vi "Find Subcrystal.vi"(10 "Base Atom":i32, 11 "Atomic Structure":T1={"Structure Name"="Gamm8", "Lattice vector a"=[4.675927601962877, 0.0, 0.0], "Lattice vector b"=[0.0, 8.100295396595834, -6.14689389815e-05], "Lattice vector c"=[0.0, -8.67870405793e-05, 11.452598090719311], "Atoms Array"=[{"Atom Name"="Cd", "Positions (Direct)"=[[0.0, 2.2797955771e-06, 0.2499966378910753], [0.5000009999999975, 0.5000032797955746, 0.2499966378910753], [0.0, 0.3333362797955778, 0.583330637891076], [0.5000009999999975, 0.8333372797955753, 0.583330637891076], [0.5000009999999975, 0.1666692797955739, 0.9166636378910721], [0.0, 0.6666702797955785, 0.9166636378910721]], "Positions (Cartesian)"=[[0.0, -3.2294507389786483e-06, 2.863111017657439], [2.3379684769090283, 4.050152569142555, 2.8630802831264797], [0.0, 2.700071707206758, 6.680630859941972], [2.3379684769090283, 6.750227505800051, 6.6806001254110114], [2.3379684769090283, 1.349990845357691, 10.49816998415932], [0.0, 5.400146643951042, 10.49813924962836]]}, {"Atom Name"="Te", "Positions (Direct)"=[[0.0, 0.3333317202044236, 0.3333363621089279], [0.5000009999999975, 0.8333327202044211, 0.3333363621089279], [0.5000009999999975, 0.1666647202044197, 0.6666703621089215], [0.0, 0.6666657202044243, 0.6666703621089215], [0.0, -2.2797955771e-06, 3.3621089247e-06], [0.5000009999999975, 0.4999987202044204, 3.3621089247e-06]], "Positions (Cartesian)"=[[0.0, 2.700056469434878, 3.8175468947088587], [2.3379684769090283, 6.7502122680281715, 3.8175161601778993], [2.3379684769090283, 1.3499756074990243, 7.635097471524269], [0.0, 5.400131406092375, 7.63506673699331], [0.0, -1.8467309405846353e-05, 3.850502238842479e-05], [2.3379684769090283, 4.050137331283887, 7.770491428735963e-06]]}], "# of atoms"=12} {"Atoms Array"."Positions (Cartesian)" format="%#_4f"; "Atoms Array"."Positions (Direct)" format="%#_3f"}) -> (0 "Base Atom Position (Cartesian)":dbl[](array[numeric]), 2 "Supercell Positions":dbl[][](array[numeric])=[[1.0, 0.0, 0.0], [0.0, 1.0, 0.0], [1.0, 1.0, 0.0], [-1.0, 2.0, 1.0], [0.0, 2.0, -0.0]], 3 "Subcrystal":T1={"Structure Name"="Gamm8 Subcrystal", "Lattice vector a"=[2.3379684769090283, 4.050155798593294, -3.073453095936429e-05], "Lattice vector b"=[0.0, 2.7000749366574968, 3.8175198422845327], "Lattice vector c"=[4.675927601962877, 0.0, 0.0], "Atoms Array"=[{"Atom Name"="Cd", "Positions (Direct)"=[[0.0, 2.2797955771e-06, 0.2499966378910753]], "Positions (Cartesian)"=[[0.0, -3.2294507389786483e-06, 2.863111017657439]]}, {"Atom Name"="Te", "Positions (Direct)"=[[0.0, -2.2797955771e-06, 3.3621089247e-06]], "Positions (Cartesian)"=[[0.0, -1.5237858666867705e-05, -2.8630725126350507]]}], "# of atoms"=2} {"Atoms Array"."Positions (Cartesian)" format="%#_4f"; "Atoms Array"."Positions (Direct)" format="%#_4f"})   [LabVIEW 2010]
uses:
  <vilib>/Analysis/baseanly.llb/Real Inverse Matrix.vi
  <vilib>/Analysis/baseanly.llb/A x Vector.vi
  <vilib>/Analysis/_algsub.llb/Real Vector Norm.vi
  <vilib>/Analysis/NI_AALPro.lvlib
  <vilib>/Analysis/NI_AALBase.lvlib
panel:
  out "norm":dbl
  out "A x Vector 2":dbl[][](array[numeric])
  out "Remaining Indicies":i32[](array[numeric])
  out "A x Vector":dbl[][](array[numeric])
  out "Recovered Positions":dbl[][](array[numeric])=[[0.33811863359999994, 1.0281858879, 1.8934606114], [4.9201686336, 1.0281858879, 1.8934606114], [2.629143633599999, 4.9963608879, 1.8934606114], [7.2111936336, 4.9963608879, 1.8934606114], [2.6155716014999992, 2.34227878455, 5.7830199243000004], [7.1976216015, 2.34227878455, 5.7830199243000004], [0.32454660149999826, 6.310453784549999, 5.7830199243000004], [4.906596601499999, 6.310453784549999, 5.7830199243000004]]
  in  "Integer Threshold":dbl=0.001
  out "Atoms Array":T2(array[cluster])=[{"Atom Name"="", "Positions (Direct)"=[[0.036896, 0.129554, 0.035254], [0.536896, 0.129554, 0.035254], [0.286896, 0.629554, 0.035254], [0.786896, 0.629554, 0.035254], [0.285415, 0.295133, 0.107673], [0.785415, 0.295133, 0.107673], [0.035415, 0.795133, 0.107673], [0.535415, 0.795133, 0.107673], [0.033615, 0.463308, 0.180101], [0.533615, 0.463308, 0.180101], [0.283615, 0.963308, 0.180101], [0.783615, 0.963308, 0.180101], [0.030844, 0.131453, 0.252535], [0.530844, 0.131453, 0.252535], [0.280844, 0.631453, 0.252535], [0.780844, 0.631453, 0.252535], [0.278379, 0.302058, 0.324923], [0.778379, 0.302058, 0.324923], [0.028379, 0.802058, 0.324923], [0.528379, 0.802058, 0.324923], [0.031198, 0.471844, 0.397363], [0.531198, 0.471844, 0.397363], [0.281198, 0.971844, 0.397363], [0.781198, 0.971844, 0.397363], [0.03247, 0.140643, 0.469814], [0.53247, 0.140643, 0.469814], [0.28247, 0.640643, 0.469814], [0.78247, 0.640643, 0.469814], [0.284308, 0.303948, 0.542263], [0.784308, 0.303948, 0.542263], [0.034308, 0.803948, 0.542263], [0.534308, 0.803948, 0.542263], [0.035944, 0.468219, 0.614701], [0.535944, 0.468219, 0.614701], [0.285944, 0.968219, 0.614701], [0.785944, 0.968219, 0.614701], [0.037813, 0.131858, 0.687216], [0.537813, 0.131858, 0.687216], [0.787813, 0.631858, 0.687216], [0.287813, 0.631858, 0.687216], [0.038238, 0.463759, 0.759817], [0.538238, 0.463759, 0.759817], [0.288238, 0.963758, 0.759817], [0.788238, 0.963758, 0.759817], [0.038639, 0.130134, 0.831025], [0.538639, 0.130134, 0.831025], [0.288639, 0.630134, 0.831025], [0.788639, 0.630134, 0.831025], [0.285712, 0.295024, 0.89873], [0.785712, 0.295024, 0.89873], [0.035712, 0.795024, 0.89873], [0.535712, 0.795024, 0.89873], [0.032596, 0.464879, 0.966384], [0.532596, 0.464879, 0.966384], [0.282596, 0.964879, 0.966384], [0.782596, 0.964879, 0.966384]], "Positions (Cartesian)"=[[0.33811863359999994, 1.0281858879, 1.8934606114], [4.9201686336, 1.0281858879, 1.8934606114], [2.6291436335999996, 4.9963608879, 1.8934606114], [7.2111936336, 4.9963608879, 1.8934606114], [2.6155716014999997, 2.34227878455, 5.7830199243000004], [7.197621601499999, 2.34227878455, 5.7830199243000004], [0.3245466015, 6.31045378455, 5.7830199243000004], [4.9065966014999995, 6.31045378455, 5.7830199243000004], [0.30805122149999997, 3.6769744458, 9.673062619100001], [4.890101221499999, 3.6769744458, 9.673062619100001], [2.5990762215, 7.6451494458, 9.673062619100001], [7.1811262215, 7.6451494458, 9.673062619100001], [0.2826575004, 1.04325701655, 13.5634275685], [4.8647075004, 1.04325701655, 13.5634275685], [2.5736825004, 5.011432016550001, 13.5634275685], [7.155732500399999, 5.011432016550001, 13.5634275685], [2.5510929938999998, 2.3972380083, 17.4513218993], [7.1331429939, 2.3972380083, 17.4513218993], [0.2600679939, 6.3654130083, 17.4513218993], [4.8421179939000005, 6.3654130083, 17.4513218993], [0.28590159179999997, 3.7447191294, 21.3420091033], [4.867951591799999, 3.7447191294, 21.3420091033], [2.5769265918, 7.7128941294, 21.3420091033], [7.158976591799999, 7.7128941294, 21.3420091033], [0.29755832699999996, 1.11619207305, 25.2332871074], [4.879608327, 1.11619207305, 25.2332871074], [2.588583327, 5.08436707305, 25.2332871074], [7.170633327, 5.08436707305, 25.2332871074], [2.6054269428, 2.4122377098, 29.124457693300002], [7.1874769428, 2.4122377098, 29.124457693300002], [0.31440194279999994, 6.3804127098, 29.124457693300002], [4.8964519428, 6.3804127098, 29.124457693300002], [0.32939441039999995, 3.71594986065, 33.0150374791], [4.9114444104, 3.71594986065, 33.0150374791], [2.6204194104, 7.684124860650001, 33.0150374791], [7.202469410399999, 7.684124860650001, 33.0150374791], [0.3465221133, 1.0464712383, 36.909752865600005], [4.9285721133, 1.0464712383, 36.909752865600005], [7.2195971133, 5.0146462383, 36.909752865600005], [2.6375471132999997, 5.0146462383, 36.909752865600005], [0.3504168558, 3.6805537396499997, 40.809087234699994], [4.9324668557999995, 3.6805537396499997, 40.809087234699994], [2.6414418557999997, 7.6487208033, 40.809087234699994], [7.2234918558, 7.6487208033, 40.809087234699994], [0.35409165989999997, 1.0327889709, 44.6336048275], [4.9361416599, 1.0327889709, 44.6336048275], [2.6451166599, 5.0009639709, 44.6336048275], [7.227166659899999, 5.0009639709, 44.6336048275], [2.6182933392, 2.3414137224, 48.269979443000004], [7.200343339199999, 2.3414137224, 48.269979443000004], [0.3272683392, 6.3095887224, 48.269979443000004], [4.9093183391999995, 6.3095887224, 48.269979443000004], [0.29871300359999997, 3.6894424516499997, 51.9036148944], [4.880763003599999, 3.6894424516499997, 51.9036148944], [2.5897380036, 7.65761745165, 51.9036148944], [7.171788003599999, 7.65761745165, 51.9036148944]]}, {"Atom Name"="", "Positions (Direct)"=[[0.286795, 0.296109, 0.054458], [0.786795, 0.296109, 0.054458], [0.036795, 0.796109, 0.054458], [0.536795, 0.796109, 0.054458], [0.035258, 0.462031, 0.126878], [0.535258, 0.462031, 0.126878], [0.285258, 0.962031, 0.126878], [0.785258, 0.962031, 0.126878], [0.033445, 0.130094, 0.199309], [0.533445, 0.130094, 0.199309], [0.283445, 0.630094, 0.199309], [0.783445, 0.630094, 0.199309], [0.280766, 0.298203, 0.27171], [0.780766, 0.298203, 0.27171], [0.030766, 0.798203, 0.27171], [0.530766, 0.798203, 0.27171], [0.028505, 0.468822, 0.344121], [0.528505, 0.468822, 0.344121], [0.278505, 0.968822, 0.344121], [0.778505, 0.968822, 0.344121], [0.03126, 0.138635, 0.416572], [0.53126, 0.138635, 0.416572], [0.28126, 0.638635, 0.416572], [0.78126, 0.638635, 0.416572], [0.282556, 0.307128, 0.489026], [0.782556, 0.307128, 0.489026], [0.032556, 0.807128, 0.489026], [0.532556, 0.807128, 0.489026], [0.034374, 0.470438, 0.56147], [0.534374, 0.470438, 0.56147], [0.284374, 0.970438, 0.56147], [0.784374, 0.970438, 0.56147], [0.035964, 0.134698, 0.633895], [0.535964, 0.134698, 0.633895], [0.285964, 0.634698, 0.633895], [0.785964, 0.634698, 0.633895], [0.037794, 0.465111, 0.706493], [0.537794, 0.465111, 0.706493], [0.787794, 0.965111, 0.706493], [0.287794, 0.965111, 0.706493], [0.038181, 0.130274, 0.779081], [0.538181, 0.130274, 0.779081], [0.288181, 0.630273, 0.779081], [0.788181, 0.630273, 0.779081], [0.288548, 0.296604, 0.847022], [0.788548, 0.296604, 0.847022], [0.038548, 0.796604, 0.847022], [0.538548, 0.796604, 0.847022], [0.035661, 0.461866, 0.914714], [0.535661, 0.461866, 0.914714], [0.285661, 0.961866, 0.914714], [0.785661, 0.961866, 0.914714], [0.032517, 0.131341, 0.982331], [0.532517, 0.131341, 0.982331], [0.282517, 0.631341, 0.982331], [0.782517, 0.631341, 0.982331]], "Positions (Cartesian)"=[[2.6282180595, 2.35002466215, 2.9248901678], [7.2102680595, 2.35002466215, 2.9248901678], [0.3371930595, 6.31819966215, 2.9248901678], [4.9192430595, 6.31819966215, 2.9248901678], [0.32310783779999996, 3.66683972685, 6.814503189799999], [4.9051578378, 3.66683972685, 6.814503189799999], [2.6141328378, 7.63501472685, 6.814503189799999], [7.1961828377999995, 7.63501472685, 6.814503189799999], [0.3064933245, 1.0324715168999998, 10.704707011899998], [4.8885433245, 1.0324715168999998, 10.704707011899998], [2.5975183244999998, 5.000646516900001, 10.704707011899998], [7.179568324499999, 5.000646516900001, 10.704707011899998], [2.5729677006, 2.36664337905, 14.593299561], [7.155017700599999, 2.36664337905, 14.593299561], [0.2819427006, 6.33481837905, 14.593299561], [4.863992700599999, 6.33481837905, 14.593299561], [0.2612226705, 3.7207354797, 18.4824292011], [4.843272670499999, 3.7207354797, 18.4824292011], [2.5522476705, 7.6889104797, 18.4824292011], [7.1342976705, 7.6889104797, 18.4824292011], [0.286469766, 1.1002558822500002, 22.3737072052], [4.8685197659999995, 1.1002558822500002, 22.3737072052], [2.577494766, 5.0684308822499995, 22.3737072052], [7.159544765999999, 5.0684308822499995, 22.3737072052], [2.5893714396, 2.4374753028000002, 26.2651463366], [7.1714214396, 2.4374753028000002, 26.2651463366], [0.2983464396, 6.4056503028, 26.2651463366], [4.8803964396, 6.4056503028, 26.2651463366], [0.3150067734, 3.7335606213, 30.156048377], [4.8970567734, 3.7335606213, 30.156048377], [2.6060317734, 7.7017356213, 30.156048377], [7.1880817733999995, 7.7017356213, 30.156048377], [0.3295776924, 1.0690104723, 34.045929944499996], [4.9116276924, 1.0690104723, 34.045929944499996], [2.6206026924, 5.0371854723, 34.045929944499996], [7.202652692399999, 5.0371854723, 34.045929944499996], [0.3463479954, 3.69128368485, 37.9451031863], [4.928397995399999, 3.69128368485, 37.9451031863], [7.2194229953999995, 7.659458684850001, 37.9451031863], [2.6373729954, 7.659458684850001, 37.9451031863], [0.34989450209999995, 1.0339000599000001, 41.843739337100004], [4.9319445020999995, 1.0339000599000001, 41.843739337100004], [2.6409195021, 5.00206712355, 41.843739337100004], [7.2229695021, 5.00206712355, 41.843739337100004], [2.6442827268, 2.3539531553999997, 45.4927893002], [7.2263327268, 2.3539531553999997, 45.4927893002], [0.35325772679999995, 6.3221281554, 45.4927893002], [4.9353077268, 6.3221281554, 45.4927893002], [0.3268009701, 3.6655302291, 49.1284656974], [4.9088509701000005, 3.6655302291, 49.1284656974], [2.6178259700999997, 7.6337052291, 49.1284656974], [7.1998759701, 7.6337052291, 49.1284656974], [0.29798903969999996, 1.04236814535, 52.760113912099996], [4.8800390397, 1.04236814535, 52.760113912099996], [2.5890140397, 5.010543145350001, 52.760113912099996], [7.1710640397, 5.010543145350001, 52.760113912099996]]}]
  # "Need not be equal since the Cd and Te aren't paired"
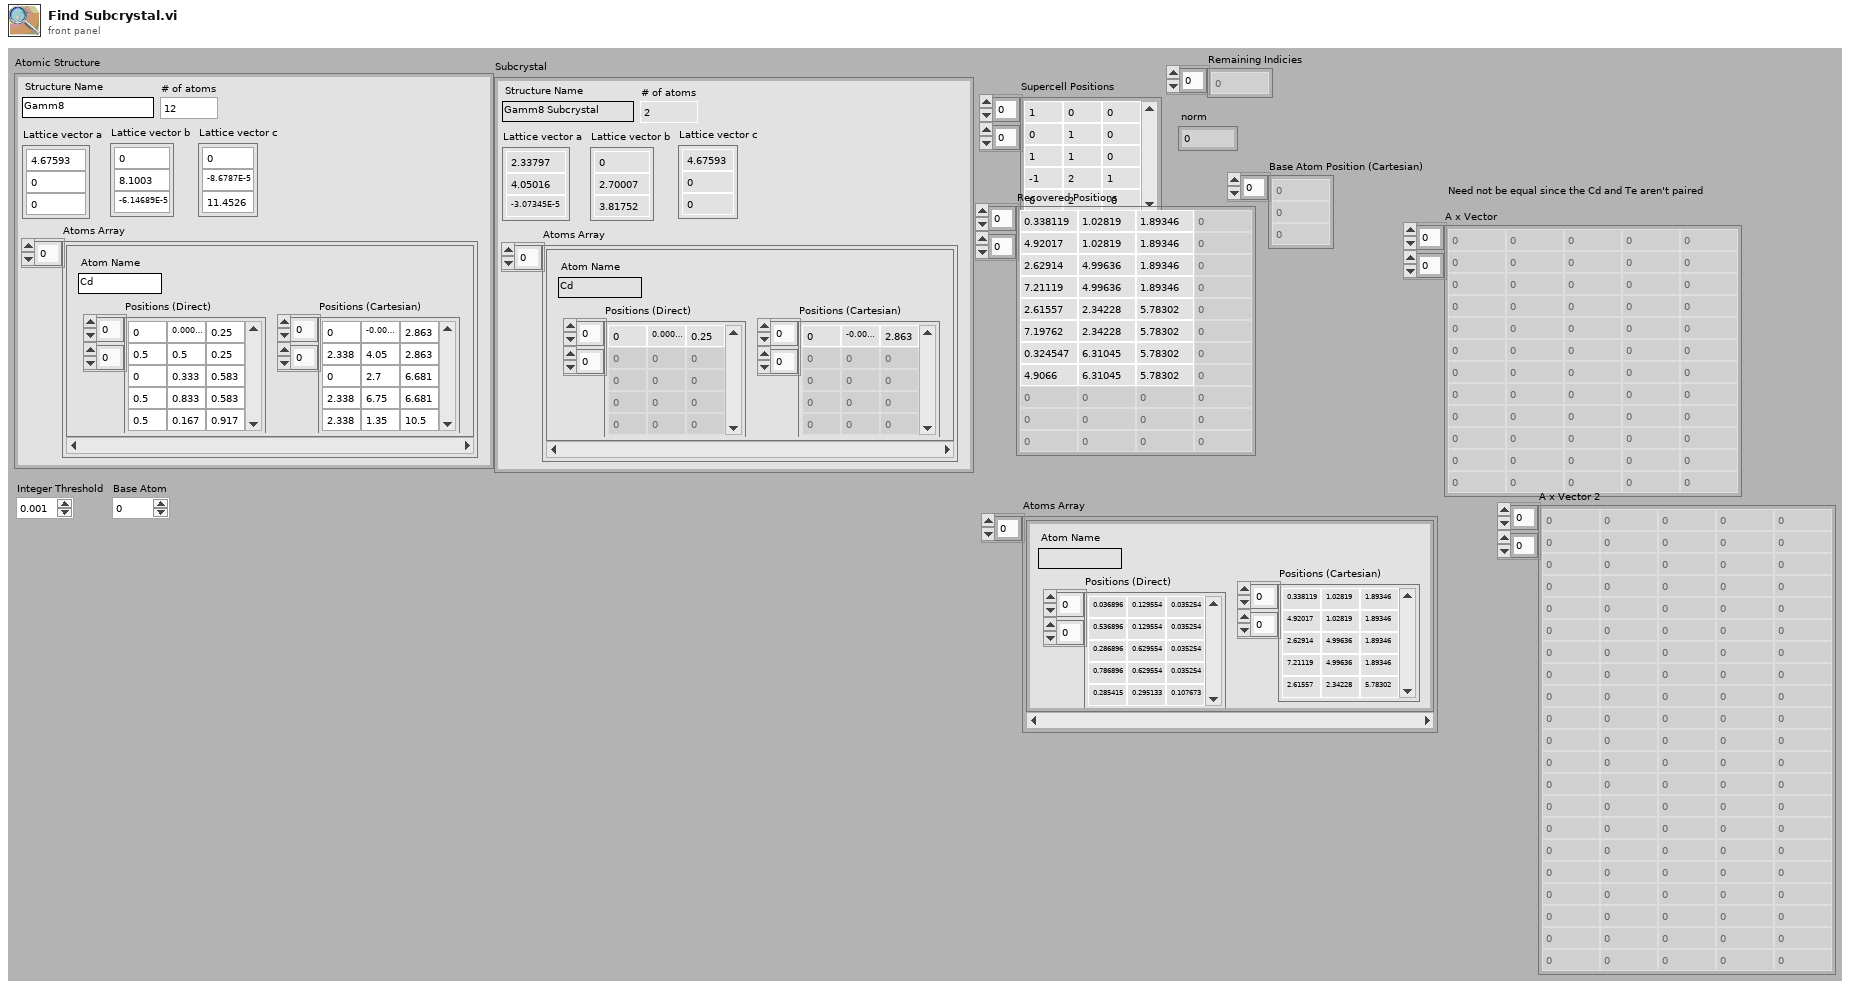
[diagram p1: front panel]
types:
  T1 = cluster{"Structure Name":string, "Lattice vector a":dbl[], "Lattice vector b":dbl[], "Lattice vector c":dbl[], "Atoms Array":cluster{"Atom Name":string, "Positions (Direct)":dbl[][], "Positions (Cartesian)":dbl[][]}[], "# of atoms":i32}
  T2 = cluster{"Atom Name":string, "Positions (Direct)":dbl[][], "Positions (Cartesian)":dbl[][]}[]
  T3 = cluster{"Atom Name":string, "Positions (Direct)":dbl[][], "Positions (Cartesian)":dbl[][]}
  T4 = typedef "NI_Matrix.lvlib/RealMatrix.ctl" = dbl[][]
  T5 = cluster{string, dbl[], dbl[], dbl[], cluster{"Atom Name":string, dbl[][], dbl[][]}[], "index (row)":i32}
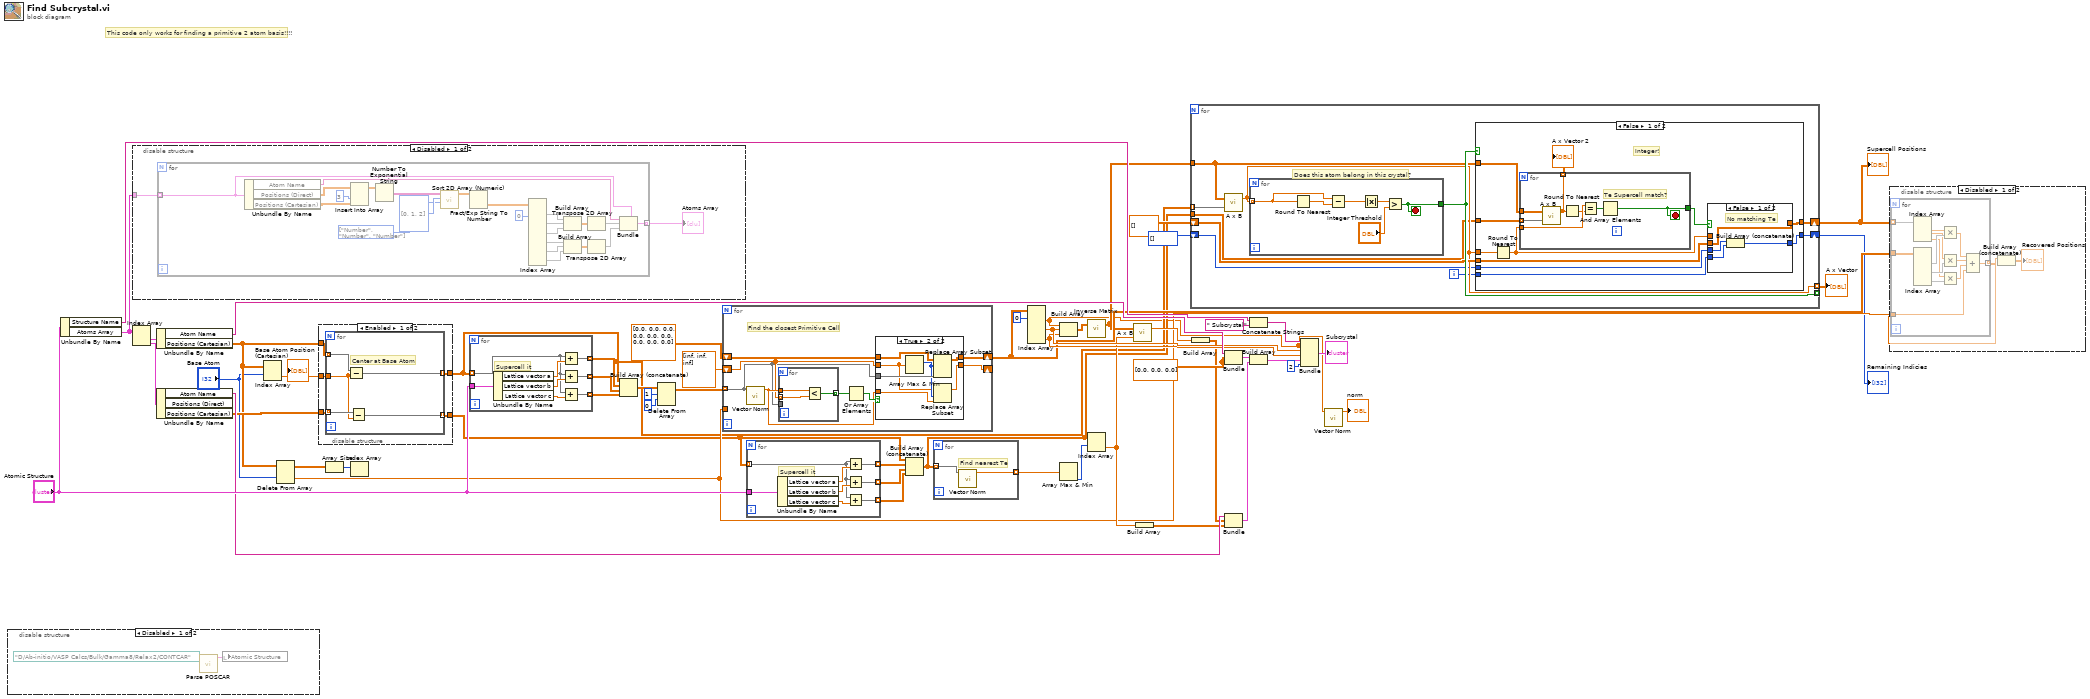
[diagram p0: block diagram]
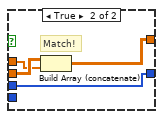
[diagram p5: hidden frame]
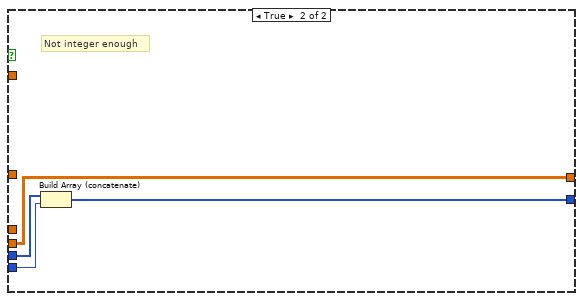
[diagram p6: hidden frame]
diagram:
  w22 = dbl[][] [[0.0, 0.0, 0.0]]
  # "This code only works for finding a primitive 2 atom basis!!!!"
  n1 = disable-structure shown="Disabled" {
    frame Disabled {
      n2 = call "Parse POSCAR.vi"("POSCAR File"=path "D:/Ab-initio/VASP Calcs/Bulk/Gamma8/Relax2/CONTCAR") -> ("Structure"=w58:T1)  [unwired: 7 in, 3 out]
      n3 = local write "Atomic Structure"(w58) -> ()
    }
    frame Enabled {
    }
  }
  n4 = Unbundle By Name("Atomic Structure") -> ("Structure Name"=w53:string, "Atoms Array"=w56:T2)
  n5 = disable-structure shown="Disabled" {
    disable-tunnel: w56 -> [w59 _]
    frame Disabled {
      n6 = for {
        tunnel: w59 -> [w61] mode=indexing
        tunnel: [w71] -> w60 mode=indexing
        w82 = enum16{"String", "Number", "Date-Time"}[] [enum."Number", enum."Number", enum."Number"] items=["String", "Number", "Date-Time"] ("Sort by Datatype Array")
        n7 = Unbundle By Name(w61) -> ("Atom Name"=w72:string, "Positions (Direct)"=w70:dbl[][], "Positions (Cartesian)"=w69:dbl[][])
        n8 = Insert Into Array(array=w70, index (col)=3 ("disabled index (col)"), new element=w69) -> (w67:dbl[][])  [unwired: 1 in]
        n9 = Number To Exponential String(number=w67) -> (E-format string=w81:string[][])  [unwired: 3 in]
        n10 = call "Sort 2D Array (Numeric).vi"(9:w82, "Sort by Cols"=i32[] [0, 1, 2], "Input Array"=w81) -> ("Output Array"=w80:dbl[][])  [unwired: 8 in]
        n11 = Fract/Exp String To Number(string=w80) -> (number=w66:dbl[][])  [unwired: 3 in, 1 out]
        n12 = Index Array(array=w66, index (col) #1=0 ("disabled index (col)")) -> (element #1=w78:dbl[], element #2=w77:dbl[], element #3=w76:dbl[], element #4=w75:dbl[], element #5=w74:dbl[], element #6=w73:dbl[])  [unwired: 11 in]
        n13 = Build Array(w78, w77, w76) -> (w65:dbl[][])
        n14 = Build Array(w75, w74, w73) -> (w63:dbl[][])
        n15 = Transpose 2D Array(2D array=w65) -> (transposed array=w64:dbl[][])
        n16 = Transpose 2D Array(2D array=w63) -> (transposed array=w62:dbl[][])
        n17 = Bundle(cluster=w61, "Atom Name"=w72, "Positions (Direct)"=w64, "Positions (Cartesian)"=w62) -> (w71:T3)
      }
      "Atoms Array" <- w60
    }
    frame Enabled {
    }
  }
  n18 = Index Array(array=w56) -> (element #1=w55:T3, element #2=w51:T3)  [unwired: 2 in]
  n19 = Unbundle By Name(w55) -> ("Atom Name"=w52:string, "Positions (Cartesian)"=w14:dbl[][])
  n20 = Unbundle By Name(w51) -> ("Atom Name"=w50:string, "Positions (Cartesian)"=w15:dbl[][])  [unwired: 1 out]
  n21 = Index Array(array=w14, index (row)="Base Atom") -> (element=w12:dbl[])  [unwired: 1 in]
  "Base Atom Position (Cartesian)" <- w12
  n22 = Delete From Array(array=w14, index (row)="Base Atom") -> (deleted portion=w16:dbl[], array with subset deleted=w31:dbl[][])  [unwired: 2 in]
  n23 = disable-structure shown="Enabled" {
    disable-tunnel: w15 -> [w88 w94]
    disable-tunnel: w14 -> [w87 w95]
    disable-tunnel: w12 -> [w86 _]
    disable-tunnel: [w85 w95] -> w7
    disable-tunnel: [w84 w94] -> w6
    frame Enabled {
      n24 = for {
        tunnel: w87 -> [w93] mode=indexing
        tunnel: w86 -> [w91]
        tunnel: w88 -> [w92] mode=indexing
        tunnel: [w90] -> w84 mode=indexing
        tunnel: [w89] -> w85 mode=indexing
        # "Center at Base Atom"
        n25 = Subtract(x=w93, y=w91) -> (x-y=w89:dbl[])
        n26 = Subtract(x=w92, y=w91) -> (x-y=w90:dbl[])
      }
    }
    frame Disabled {
    }
  }
  n27 = Array Size(array=w31) -> (size(s)=w43:i32[])
  n28 = Index Array(array=w43) -> ()  [unwired: 1 in, 1 out]
  n29 = for {
    tunnel: w7 -> [w100] mode=indexing
    tunnel: "Atomic Structure" -> [w103]
    tunnel: [w98] -> w47 mode=indexing
    tunnel: [w97] -> w46 mode=indexing
    tunnel: [w96] -> w45 mode=indexing
    # "Supercell it"
    n30 = Unbundle By Name(w103) -> ("Lattice vector a"=w102:dbl[], "Lattice vector b"=w101:dbl[], "Lattice vector c"=w99:dbl[])
    n31 = Add(x=w100, y=w102) -> (x+y=w98:dbl[])
    n32 = Add(x=w100, y=w101) -> (x+y=w97:dbl[])
    n33 = Add(x=w100, y=w99) -> (x+y=w96:dbl[])
  }
  n34 = Build Array (concatenate)(w7, w47, w46, w45) -> (w11:dbl[][])
  n35 = Delete From Array(array=w11, length=1, index (row)=0) -> (array with subset deleted=w8:dbl[][])  [unwired: 1 in, 1 out]
  n36 = for {
    tunnel: w16 -> [_]
    tunnel: w8 -> [w104] mode=indexing
    shift-right: [w105] -> _
    shift-left: dbl[] [inf, inf, inf] -> [w106]
    shift-right: [w108] -> w32
    shift-left: dbl[][] [[0.0, 0.0, 0.0], [0.0, 0.0, 0.0], [0.0, 0.0, 0.0]] -> [w109]
    # "Find the closest Primitive Cell"
    n37 = call-poly <vilib>:"Vector Norm.vi"("Input Vector"=w104) -> ("norm"=w107:dbl)  [unwired: 9 in, 1 out]
    n38 = for {
      tunnel: w107 -> [w123]
      tunnel: w106 -> [w122] mode=indexing
      tunnel: w104 -> [_]
      tunnel: [w121] -> w111 mode=indexing
      n39 = Less?(x=w123, y=w122) -> (x < y?=w121:bool)
    }
    n40 = Or Array Elements(Boolean array=w111) -> (logical OR=w110:bool)
    n41 = case shown="True" w110 {
      tunnel: [w113 w120] -> w108
      tunnel: w109 -> [w113 w119]
      tunnel: w104 -> [_ w118]
      tunnel: w106 -> [w112 w114]
      tunnel: w107 -> [_ w117]
      tunnel: [w112 w116] -> w105
      frame False {
      }
      frame True {
        n42 = Array Max & Min(array=w114) -> (max index (indices)=w115:i32)  [unwired: 3 out]
        n43 = Replace Array Subset(array=w119, new element=w118, index (row)=w115) -> (w120:dbl[][])  [unwired: 1 in]
        n44 = Replace Array Subset(array=w114, new element=w117, index=w115) -> (w116:dbl[])
      }
    }
  }
  n45 = for {
    tunnel: w6 -> [w128] mode=indexing
    tunnel: "Atomic Structure" -> [w131]
    tunnel: [w126] -> w30 mode=indexing
    tunnel: [w125] -> w29 mode=indexing
    tunnel: [w124] -> w28 mode=indexing
    # "Supercell it"
    n46 = Unbundle By Name(w131) -> ("Lattice vector a"=w130:dbl[], "Lattice vector b"=w129:dbl[], "Lattice vector c"=w127:dbl[])
    n47 = Add(x=w128, y=w130) -> (x+y=w126:dbl[])
    n48 = Add(x=w128, y=w129) -> (x+y=w125:dbl[])
    n49 = Add(x=w128, y=w127) -> (x+y=w124:dbl[])
  }
  n50 = Build Array (concatenate)(w6, w30, w29, w28) -> (w5:dbl[][])
  n51 = for {
    tunnel: w5 -> [w132] mode=indexing
    tunnel: [w133] -> w27 mode=indexing
    # "Find nearest Te"
    n52 = call-poly <vilib>:"Vector Norm.vi"("Input Vector"=w132) -> ("norm"=w133:dbl)  [unwired: 9 in, 1 out]
  }
  n53 = Index Array(array=w32, index (row) #1=0 ("index (row)")) -> (element #1=w2:dbl[], element #2=w34:dbl[], element #3=w33:dbl[])  [unwired: 5 in]
  n54 = Build Array(w2, w34, w33) -> (w21:T4)
  n55 = Array Max & Min(array=w27) -> (min index (indices)=w25:i32)  [unwired: 3 out]
  n56 = call-poly <vilib>:"Inverse Matrix.vi"("Input Matrix"=w21) -> ("Inverse Matrix"=w17:T4)  [unwired: 1 in, 1 out]
  n57 = Index Array(array=w5, index (row)=w25) -> (element=w20:dbl[])  [unwired: 1 in]
  n58 = call-poly <vilib>:"A x B.vi"("Vector"=w20, "A"=w17) -> ("A x Vector"=w19:dbl[])  [unwired: 1 out]
  n59 = Build Array(w20) -> (w26:dbl[][])
  n60 = for {
    tunnel: w17 -> [w137]
    shift-right: [w143] -> w35
    shift-left: dbl[][] [] -> [w141]
    tunnel: [w142] -> _ mode=indexing
    tunnel: w7 -> [w140] mode=indexing
    tunnel: [w139] -> w23 mode=indexing
    tunnel: w5 -> [w138]
    shift-right: [w135] -> w3
    shift-left: i32[] [] -> [w134]
    i -> [w136]
    # "Does this atom belong in this crystal?"
    n61 = call-poly <vilib>:"A x B.vi"("Vector"=w140, "A"=w137) -> ("A x Vector"=w139:dbl[])  [unwired: 1 out]
    n62 = for {
      tunnel: [w174] -> w142
      tunnel: w139 -> [w176] mode=indexing
      stop <- w174 stop-if-true
      n63 = Round To Nearest(number=w176) -> (nearest integer value=w175:dbl)
      n64 = Subtract(x=w176, y=w175) -> (x-y=w178:dbl)
      n65 = Absolute Value(x=w178) -> (abs(x)=w179:dbl)
      n66 = Greater?(x=w179, y="Integer Threshold") -> (0:w174:bool)
    }
    n67 = case shown="False" w142 {
      tunnel: [w150 w173] -> w143
      tunnel: w141 -> [w151 w173]
      tunnel: w139 -> [w154 _]
      tunnel: w138 -> [w153 _]
      tunnel: w137 -> [w152 _]
      tunnel: w136 -> [w148 w171]
      tunnel: [w147 w170] -> w135
      tunnel: w134 -> [w146 w172]
      frame False {
        # "Integer!"
        n68 = Round To Nearest(number=w154) -> (nearest integer value=w149:dbl[])
        n69 = for {
          tunnel: w149 -> [w169]
          tunnel: w153 -> [w168] mode=indexing
          tunnel: w152 -> [w167]
          tunnel: [w164] -> w145
          tunnel: [w163] -> w144 mode=indexing
          stop <- w164 stop-if-true
          # "Te Supercell match?"
          n70 = call-poly <vilib>:"A x B.vi"("Vector"=w168, "A"=w167) -> ("A x Vector"=w163:dbl[])  [unwired: 1 out]
          n71 = Round To Nearest(number=w163) -> (nearest integer value=w166:dbl[])
          n72 = Equal?(x=w169, y=w166) -> (x = y?=w165:bool[])
          n73 = And Array Elements(Boolean array=w165) -> (logical AND=w164:bool)
        }
        "A x Vector 2" <- w144
        n74 = case shown="False" w145 {
          tunnel: w151 -> [w158 w162]
          tunnel: [w158 w161] -> w150
          tunnel: w149 -> [_ w160]
          tunnel: w148 -> [w157 _]
          tunnel: [w156 w159] -> w147
          tunnel: w146 -> [w155 w159]
          frame False {
            # "No matching Te"
            n75 = Build Array (concatenate)(w155, w157) -> (w156:i32[])
          }
          frame True {
            # "Match!"
            n76 = Build Array (concatenate)(w162, w160) -> (w161:dbl[][])
          }
        }
      }
      frame True {
        # "Not integer enough"
        n77 = Build Array (concatenate)(w172, w171) -> (w170:i32[])
      }
    }
  }
  "Supercell Positions" <- w35
  "A x Vector" <- w23
  "Remaining Indicies" <- w3
  n78 = Build Array(w19) -> (w18:dbl[][])
  n79 = Bundle("Atom Name"=w52, w22, w22) -> (w39:cluster{"Atom Name":string, dbl[][], dbl[][]})  [unwired: 1 in]
  n80 = Bundle("Atom Name"=w50, w18, w26) -> (w24:cluster{"Atom Name":string, dbl[][], dbl[][]})  [unwired: 1 in]
  n81 = Concatenate Strings(w53, " Subcrystal" ("string")) -> (w41:string)
  n82 = Build Array(w39, w24) -> (w38:cluster{"Atom Name":string, dbl[][], dbl[][]}[])
  n83 = Bundle(w41, w2, w34, w33, w38, "index (row)"=2) -> (→"Subcrystal":T5)  [unwired: 1 in]
  n84 = call-poly <vilib>:"Vector Norm.vi"("Input Vector"=w2) -> ("norm"=→"norm":dbl)  [unwired: 9 in, 1 out]
  n85 = disable-structure shown="Disabled" {
    disable-tunnel: w35 -> [w184 _]
    disable-tunnel: w32 -> [w183 _]
    disable-tunnel: w16 -> [w182 _]
    frame Disabled {
      n86 = for {
        tunnel: w184 -> [w189] mode=indexing
        tunnel: w183 -> [w190]
        tunnel: [w186] -> w181 mode=indexing
        tunnel: w182 -> [w185]
        n87 = Index Array(array=w189) -> (element #1=w191:dbl, element #2=w192:dbl, element #3=w193:dbl)  [unwired: 3 in]
        n88 = Index Array(array=w190) -> (element #1=w194:dbl[], element #2=w195:dbl[], element #3=w188:dbl[])  [unwired: 6 in]
        n89 = Multiply(x=w191, y=w194) -> (x*y=w196:dbl[])
        n90 = Multiply(x=w192, y=w195) -> (x*y=w197:dbl[])
        n91 = Multiply(x=w193, y=w188) -> (x*y=w187:dbl[])
        n92 = Compound Arithmetic op=ADD(w196, w197, w187, w185) -> (w186:dbl[])
      }
      n93 = Build Array (concatenate)(w182, w181) -> (→"Recovered Positions":dbl[][])
    }
    frame Enabled {
    }
  }
